vi "main--example pop-up svg.vi"() -> ()   [LabVIEW 2021]
doc: "This VI will show an example of loading an image in as custom SVGs."
uses:
  <vilib>/addons/_TSC/TSC Pop-Up/Popup/message info--typedef.ctl
  user32.dll
  Custom/SVG - One Button/SVG - One Button.lvclass
  <vilib>/addons/_TSC/TSC Pop-Up/Popup/Popup.lvclass
panel:
  in  "Close":bool
  out "header":bool
  in  "check it out":bool
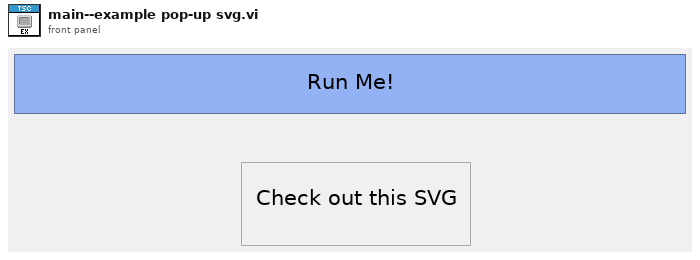
[diagram p1: front panel]
types:
  T1 = typedef "Pop-Up.lvlib/Popup.lvclass/message info--typedef.ctl" = cluster{"Message Height":i32, "Message Width":i32, "Message Location":enum16{"Top", "Bottom", "Right", "Left"}}
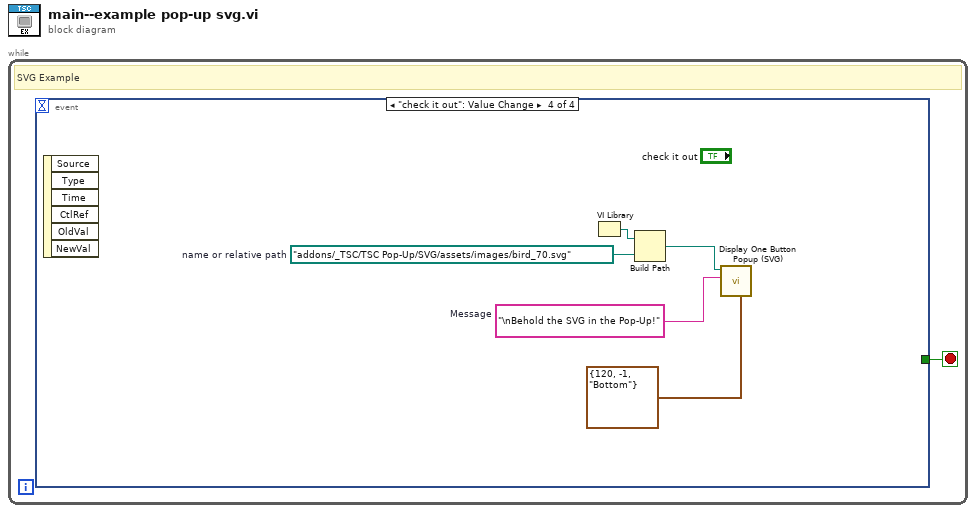
[diagram p0: block diagram]
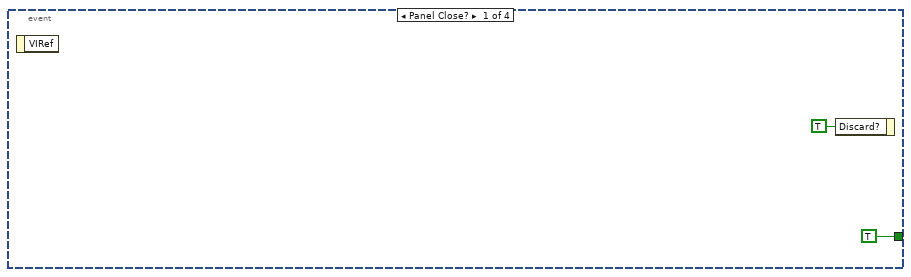
[diagram p2: hidden frame]
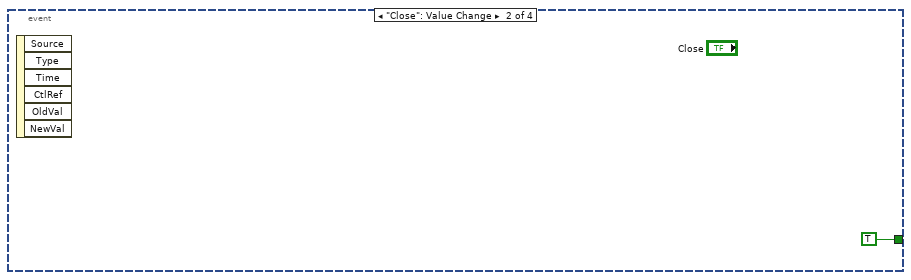
[diagram p3: hidden frame]
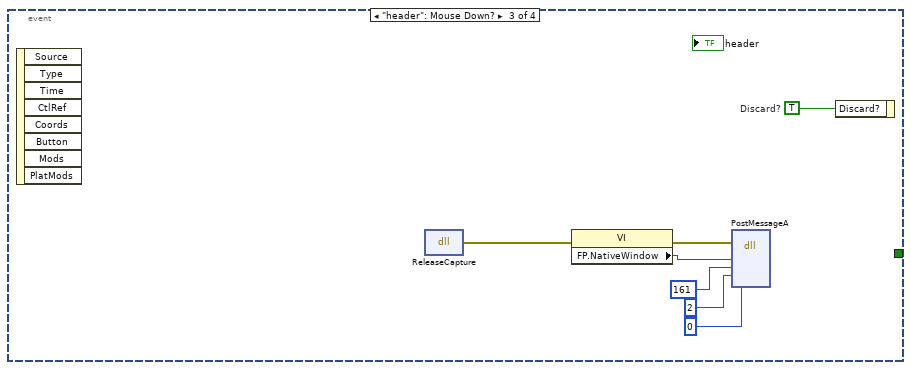
[diagram p4: hidden frame]
diagram:
  n1 = while {
    stop <- w1 stop-if-true
    # "SVG Example"
    n2 = event shown="[3] \"check it out\": Value Change" {
      selector: _ -> [_ _ _ _]
      dyn-events: _ -> [_ _ _ _]
      timeout: _ -> [_ _ _ _]
      tunnel: [TRUE TRUE _ _] -> w1
      event Panel Close? {
        n3 = event-data() -> ()  [unwired: 1 in, 1 out]
        n4 = event-data("Discard?"=TRUE) -> ()  [unwired: 1 in, 1 out]
      }
      event "Close": Value Change {
        n5 = event-data() -> ()  [unwired: 1 in, 6 out]
      }
      event "header": Mouse Down? {
        w11 = TRUE  # Discard?
        n6 = event-data() -> ()  [unwired: 1 in, 8 out]
        n7 = dll-call lib="user32.dll" fn="ReleaseCapture"() -> (error out=w7:errorcluster)  [unwired: 4 in, 1 out]
        n8 = property class="VI"(error in=w7) -> (error out=w6:errorcluster, "FP.NativeWindow"=w5:u64)  [unwired: 1 in, 1 out]
        n9 = dll-call lib="user32.dll" fn="PostMessageA"(error in=w6, "hWnd"=w5, "Msg"=161, "wParam"=2, "lParam"=0) -> ()  [unwired: 7 in, 2 out]
        n10 = event-data("Discard?"=w11) -> ()  [unwired: 1 in, 1 out]
      }
      event "check it out": Value Change {
        w15 = path "addons/_TSC/TSC Pop-Up/SVG/assets/images/bird_70.svg"  # name or relative path
        w14 = "\nBehold the SVG in the Pop-Up!"  # Message
        n11 = event-data() -> ()  [unwired: 1 in, 6 out]
        n12 = VI Library() -> (path=w16:path)
        n13 = Build Path(base path=w16, name or relative path=w15) -> (appended path=w12:path)
        n14 = call "Display One Button Popup (SVG).vi"("Message Size"=T1 {"Message Height"=120, "Message Width"=-1, "Message Location"=enum."Bottom"}, "Message"=w14, "Graphic"=w12) -> ()  [unwired: 8 in, 1 out]
      }
    }
  }
